vi "five digits sum.vi"   [LabVIEW 2020]
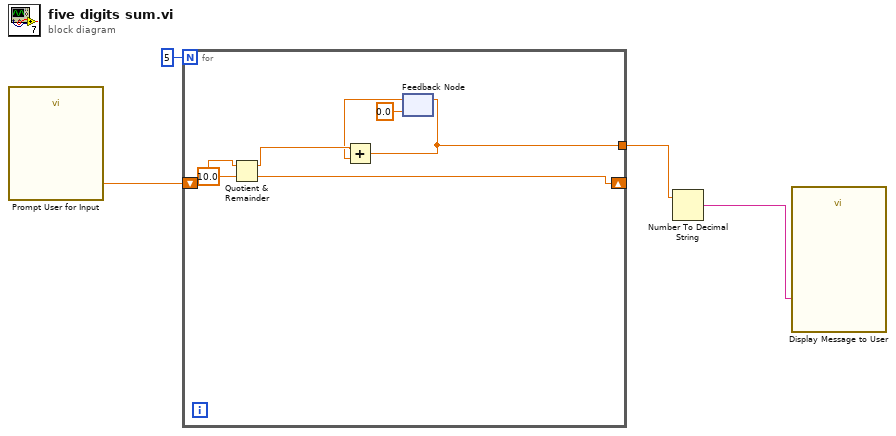
[diagram p0: block diagram]
diagram:
  n1 = call "Prompt User for Input"() -> ("Number"=w3:dbl)  [unwired: 17 in, 2 out]
  n2 = for {
    N: 5 -> [_]
    shift-right: [w6] -> _
    shift-left: w3 -> [w10]
    tunnel: [w5] -> w2
    n3 = Quotient & Remainder(x=w10, y=10.0) -> (x-y*floor(x/y)=w11:dbl, floor(x/y)=w6:dbl)
    n4 = feedback #1(0.0) -> (w9:dbl)
    n5 = Add(x=w11, y=w9) -> (x+y=w5:dbl)
    n6 = feedback-in #1(w5) -> ()
  }
  n7 = Number To Decimal String(number=w2) -> (decimal integer string=w1:string)  [unwired: 1 in]
  n8 = call "Display Message to User"("Message"=w1) -> ()  [unwired: 9 in, 2 out]
